vi "RD Digital Out Counter Init Set.vi"(7 "counter":u32, 8 "error in (no error)":errorcluster caption="错误输入（无错误）", 9 "initlevel":i32, 10 "ch":i32, 11 "handle":u64) -> (0 "error out":errorcluster caption="错误输出", 2 "function return":i32, 3 "handle out":u64)   [LabVIEW 2018, in "InstrumentsPlayground.lvlib"]
doc: "CLIFFAPI int CliffDigitalOutCounterInitSet(FT_HANDLE handle,int ch,int initlevel,uint counter);\nch: 0x0001 : ch1 ; 0x0002 : ch2 ; .... 0x8000 :ch16\ninitlevel:0 : low level ,1 : high level.\ncounter: 1for 5ns. max :0xFFFFFFFF"
uses:
  InstrumentsPlayground.lvlib
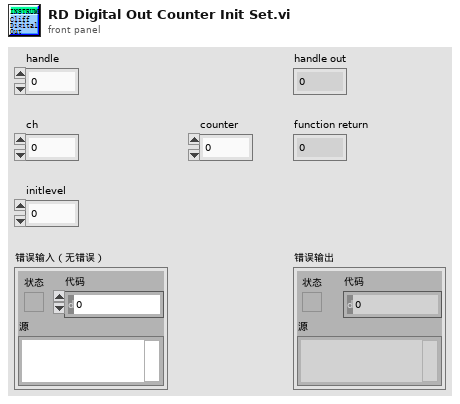
[diagram p1: front panel]
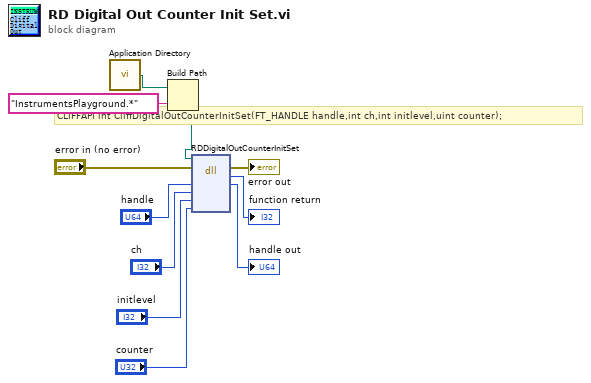
[diagram p0: block diagram]
diagram:
  # "CLIFFAPI int CliffDigitalOutCounterInitSet(FT_HANDLE handle,int ch,int initlevel,uint counter);"
  n1 = call <vilib>:"Application Directory.vi"() -> ("Application Directory"=w2:path)
  n2 = Build Path(base path=w2, name or relative path="InstrumentsPlayground.*" ("名称或相对路径")) -> (appended path=w1:path)
  n3 = dll-call lib="E:/work/YZCourse_Xtext/Cliff/API/LabVIEW lib/InstrumentsPlayground.*" fn="RDDigitalOutCounterInitSet"(path in=w1, error in="error in (no error)", "handle"="handle", "ch"="ch", "initlevel"="initlevel", "counter"="counter") -> (error out=→"error out":errorcluster, "返回类型"=→"function return":i32, "handle"=→"handle out":u64)  [unwired: 4 in, 1 out]
